vi "Autonomous Independent.vi"   [LabVIEW 2017] (continued)
                          n864 = call "PID Distance.vi"("Distance"=26.0, "Angle"=w3022, "RightEncoder"=w3027, "LeftEncoder"=w3028, "GyroDevRef"=w3029, "RobotDriveDevRef"=w3030) -> ("RightEncoder 2"=w3023:T11, "LeftEncoder 2"=w3024:T11, "GyroDevRef 2"=w3025:T8, "RobotDriveDevRef 2"=w3026:T1)  [unwired: 2 in]
                        }
                        frame #4 {
                          n865 = global write "Robot Global Data.vi" "Current State"(TRUE ("Current State")) -> ()
                          n866 = Wait (ms)(milliseconds to wait=u32 500) -> ()  [unwired: 1 out]
                        }
                        frame #5 {
                          n867 = global read "Robot Global Data.vi" "Axes"() -> (w3043:dbl[])
                          n868 = global write "Robot Global Data.vi" "Lift_Position"(2.0) -> ()
                          n869 = Wait (ms)(milliseconds to wait=u32 250) -> ()  [unwired: 1 out]
                          n870 = Array To Cluster(array=w3043) -> (cluster=w3042:T15)
                          n871 = Bundle By Name(cluster=w3042, "Axes[1]"=-1.0) -> (w3040:T15)
                          n872 = Cluster To Array(cluster=w3040) -> (array=w3039:dbl[])
                          n873 = global write "Robot Global Data.vi" "Axes"(w3039) -> ()
                        }
                        frame #6 {
                          n874 = global read "Robot Global Data.vi" "Tracked Angle"() -> (w3049:dbl)
                          n875 = call "PID Distance.vi"("Distance"=40.0, "Angle"=w3049, "RightEncoder"=w3050, "LeftEncoder"=w3053, "GyroDevRef"=w3052, "RobotDriveDevRef"=w3051) -> ()  [unwired: 2 in, 4 out]
                        }
                        frame #7 {
                          n876 = global read "Robot Global Data.vi" "Axes"() -> (w3060:dbl[])
                          n877 = Wait (ms)(milliseconds to wait=u32 250) -> ()  [unwired: 1 out]
                          n878 = Array To Cluster(array=w3060) -> (cluster=w3059:T15)
                          n879 = Bundle By Name(cluster=w3059, "Axes[1]"=1.0) -> (w3057:T15)
                          n880 = Cluster To Array(cluster=w3057) -> (array=w3056:dbl[])
                          n881 = global write "Robot Global Data.vi" "Axes"(w3056) -> ()
                        }
                        frame #8 {
                          n882 = global write "Robot Global Data.vi" "Current State"(FALSE ("Current State")) -> ()
                        }
                      }
                    }
                    frame Default {
                    }
                  }
                }
              }
            }
            frame "L" {
              n883 = flat-sequence {
                tunnel: [w3127] -> w3115
                tunnel: [w3126] -> w3116
                tunnel: [w3124] -> w3117
                tunnel: [w3125] -> w3118
                tunnel: w3074 -> [w3123]
                tunnel: w3073 -> [w3122]
                tunnel: w3072 -> [w3121]
                tunnel: w3071 -> [w3120]
                tunnel: [w3148] -> w3114
                tunnel: w3118 -> [w3144]
                tunnel: w3117 -> [w3145]
                tunnel: w3116 -> [w3147]
                tunnel: w3115 -> [w3149]
                tunnel: [w3146] -> w3113
                tunnel: [w3145] -> w3112
                tunnel: [w3144] -> w3111
                tunnel: w3114 -> [w3159]
                tunnel: [w3159] -> w3110
                tunnel: w3113 -> [w3158]
                tunnel: [w3158] -> w3109
                tunnel: [w3157] -> w3108
                tunnel: [w3156] -> w3107
                tunnel: w3112 -> [w3154]
                tunnel: w3111 -> [w3153]
                tunnel: w3110 -> [w3165]
                tunnel: [w3163] -> w3106
                tunnel: w3109 -> [w3164]
                tunnel: [w3162] -> w3105
                tunnel: w3108 -> [w3167]
                tunnel: w3107 -> [w3166]
                tunnel: [w3161] -> w3104
                tunnel: [w3160] -> w3103
                tunnel: w3106 -> [w3174]
                tunnel: [w3173] -> w3102
                tunnel: [w3172] -> w3101
                tunnel: w3105 -> [w3172]
                tunnel: [w3171] -> w3100
                tunnel: w3104 -> [w3171]
                tunnel: [w3170] -> w3099
                tunnel: w3103 -> [w3170]
                tunnel: [w3185] -> w3098
                tunnel: w3102 -> [w3185]
                tunnel: [w3184] -> w3097
                tunnel: w3101 -> [w3184]
                tunnel: [w3183] -> w3096
                tunnel: w3100 -> [w3183]
                tunnel: [w3182] -> w3095
                tunnel: w3099 -> [w3182]
                tunnel: w3098 -> [w3190]
                tunnel: w3097 -> [w3191]
                tunnel: [w3191] -> w3094
                tunnel: [w3190] -> w3093
                tunnel: [w3189] -> w3092
                tunnel: w3096 -> [w3189]
                tunnel: [w3188] -> w3091
                tunnel: w3095 -> [w3188]
                tunnel: [w3204] -> w3090
                tunnel: w3094 -> [w3206]
                tunnel: w3093 -> [w3205]
                tunnel: w3092 -> [w3201]
                tunnel: w3091 -> [w3200]
                tunnel: [w3199] -> w3089
                tunnel: [w3198] -> w3088
                tunnel: [w3197] -> w3087
                tunnel: w3090 -> [w3213]
                tunnel: w3089 -> [w3212]
                tunnel: [w3211] -> w3069
                tunnel: w3088 -> [w3211]
                tunnel: [w3210] -> w3067
                tunnel: w3087 -> [w3210]
                tunnel: [w3209] -> w3065
                tunnel: [w3208] -> w3063
                tunnel: w3069 -> [w3220]
                tunnel: [w3216] -> w3068
                tunnel: w3067 -> [w3219]
                tunnel: [w3215] -> w3066
                tunnel: w3065 -> [w3222]
                tunnel: [w3218] -> w3064
                tunnel: w3063 -> [w3221]
                tunnel: [w3217] -> w3062
                tunnel: w3068 -> [w3248]
                tunnel: w3066 -> [w3247]
                tunnel: [w3245] -> w3086
                tunnel: w3064 -> [w3245]
                tunnel: [w3244] -> w3085
                tunnel: w3062 -> [w3244]
                tunnel: [w3243] -> w3084
                tunnel: [w3242] -> w3083
                tunnel: w3086 -> [w3263]
                tunnel: w3085 -> [w3262]
                tunnel: w3084 -> [w3261]
                tunnel: w3083 -> [w3260]
                tunnel: [w3259] -> w3082
                tunnel: [w3258] -> w3081
                tunnel: [w3257] -> w3080
                tunnel: [w3256] -> w3079
                tunnel: [w3268] -> w3078
                tunnel: [w3265] -> w3077
                tunnel: [w3267] -> w3076
                tunnel: [w3266] -> w3075
                tunnel: w3079 -> [w3265]
                tunnel: w3080 -> [w3266]
                tunnel: w3081 -> [w3267]
                tunnel: w3082 -> [w3268]
                tunnel: w3078 -> [w3275]
                tunnel: w3077 -> [w3274]
                tunnel: w3076 -> [w3273]
                tunnel: w3075 -> [w3272]
                tunnel: w3070 -> [w3271]
                frame #0 {
                  n884 = while {
                    tunnel: [w3133] -> w3119
                    stop <- w3132 stop-if-true
                    w3136 = 100.0 ("y")
                    w3139 = 20.0 ("y")
                    n885 = Wait (ms)(milliseconds to wait=u32 10) -> ()  [unwired: 1 out]
                    n886 = global read "Robot Global Data.vi" "Distance 2"() -> (w3134:dbl)
                    n887 = global read "Robot Global Data.vi" "Distance"() -> (w3135:dbl)
                    n888 = Greater?(x=w3135, y=w3139) -> (0:w3141:bool)
                    n889 = Greater?(x=w3134, y=w3139) -> (0:w3140:bool)
                    n890 = Greater?(x=w3135, y=w3136) -> (0:w3138:bool)
                    n891 = Greater?(x=w3134, y=w3136) -> (0:w3137:bool)
                    n892 = Or(x=w3141, y=w3140) -> (x .or. y?=w3130:bool)
                    n893 = Or(x=w3138, y=w3137) -> (x .or. y?=w3132:bool)
                    n894 = global write "Robot Global Data.vi" "Raise_Mast"(w3130) -> ()
                    n895 = case shown="True" w3132 {
                      tunnel: [0.0 2.0] -> w3133
                      frame False {
                      }
                      frame True {
                      }
                    }
                  }
                  n896 = call "PID Distance.vi"("Distance"=295.0, "Angle"=-2.0, "RightEncoder"=w3120, "LeftEncoder"=w3121, "GyroDevRef"=w3122, "RobotDriveDevRef"=w3123) -> ("RightEncoder 2"=w3124:T11, "LeftEncoder 2"=w3125:T11, "GyroDevRef 2"=w3126:T8, "RobotDriveDevRef 2"=w3127:T1)  [unwired: 2 in]
                  n897 = global write "Robot Global Data.vi" "Lift_Position"(w3119) -> ()
                }
                frame #1 {
                  n898 = call "PID turning.vi"("Angle"=90.0, "GyroDevRef"=w3147, "RobotDriveDevRef"=w3149) -> ("GyroDevRef 2"=w3146:T8, "RobotDriveDevRef 2"=w3148:T1)  [unwired: 7 in]
                  n899 = global write "Robot Global Data.vi" "Lift_Position"(3.0) -> ()
                  n900 = global write "Robot Global Data.vi" "Raise_Mast"(TRUE ("Current State")) -> ()
                }
                frame #2 {
                  n901 = call <vilib>:"WPI_EncoderReset.vi"("EncoderDevRef"=w3153) -> ("EncoderDevRef"=w3156:T11)  [unwired: 9 in, 1 out]
                  n902 = Wait (ms)(milliseconds to wait=u32 100) -> ()  [unwired: 1 out]
                  n903 = call <vilib>:"WPI_EncoderReset.vi"("EncoderDevRef"=w3154) -> ("EncoderDevRef"=w3157:T11)  [unwired: 9 in, 1 out]
                }
                frame #3 {
                  n904 = call "PID Distance.vi"("Distance"=25.0, "Angle"=90.0, "RightEncoder"=w3167, "LeftEncoder"=w3166, "GyroDevRef"=w3164, "RobotDriveDevRef"=w3165) -> ("RightEncoder 2"=w3160:T11, "LeftEncoder 2"=w3161:T11, "GyroDevRef 2"=w3162:T8, "RobotDriveDevRef 2"=w3163:T1)  [unwired: 2 in]
                }
                frame #4 {
                  w3175 = 0.0 ("Left axis value")
                  n905 = global read "Robot Global Data.vi" "Axes"() -> (w3178:dbl[])
                  n906 = Wait (ms)(milliseconds to wait=u32 500) -> ()  [unwired: 1 out]
                  n907 = Array To Cluster(array=w3178) -> (cluster=w3177:T15)
                  n908 = Bundle By Name(cluster=w3177, "Axes[1]"=0.25) -> (w3180:T15)
                  n909 = Cluster To Array(cluster=w3180) -> (array=w3179:dbl[])
                  n910 = call <vilib>:"WPI_RobotDriveTankDrive.vi"("Right axis value"=w3175, "Left axis value"=w3175, "RobotDriveDevRef"=w3174) -> ("RobotDriveDevRef"=w3173:T1)  [unwired: 6 in, 2 out]
                  n911 = global write "Robot Global Data.vi" "Axes"(w3179) -> ()
                }
                frame #5 {
                  n912 = global write "Robot Global Data.vi" "Current State"(FALSE ("Current State")) -> ()
                  n913 = Wait (ms)(milliseconds to wait=u32 400) -> ()  [unwired: 1 out]
                }
                frame #6 {
                  n914 = global read "Robot Global Data.vi" "Axes"() -> (w3193:dbl[])
                  n915 = Array To Cluster(array=w3193) -> (cluster=w3192:T15)
                  n916 = Bundle By Name(cluster=w3192, "Axes[1]"=-1.0) -> (w3195:T15)
                  n917 = Cluster To Array(cluster=w3195) -> (array=w3194:dbl[])
                  n918 = global write "Robot Global Data.vi" "Axes"(w3194) -> ()
                }
                frame #7 {
                  n919 = call "PID Distance.vi"("Distance"=7.0, "Angle"=90.0, "RightEncoder"=w3200, "LeftEncoder"=w3201, "GyroDevRef"=w3206, "RobotDriveDevRef"=w3205) -> ("RightEncoder 2"=w3197:T11, "LeftEncoder 2"=w3198:T11, "GyroDevRef 2"=w3199:T8, "RobotDriveDevRef 2"=w3204:T1)  [unwired: 2 in]
                }
                frame #8 {
                  n920 = global write "Robot Global Data.vi" "Lift_Position"(1.0) -> ()
                  n921 = call "PID turning.vi"("Angle"=155.0, "GyroDevRef"=w3212, "RobotDriveDevRef"=w3213) -> ("GyroDevRef 2"=w3208:T8, "RobotDriveDevRef 2"=w3209:T1)  [unwired: 7 in]
                }
                frame #9 {
                  n922 = global read "Robot Global Data.vi" "PIXY Output"() -> (w3226:T16)
                  n923 = Unbundle By Name(w3226) -> ("SIGNATURE NUMBER"=w3225:u16)
                  n924 = global read "Robot Global Data.vi" "Cube Signature"() -> (w3224:dbl)
                  n925 = Equal?(x=w3225, y=w3224) -> (x = y?=w3223:bool)
                  n926 = case shown="False" w3223 {
                    tunnel: [w3233 w3237] -> w3215
                    tunnel: [w3232 w3238] -> w3216
                    tunnel: [w3231 w3239] -> w3217
                    tunnel: [w3235 w3240] -> w3218
                    tunnel: w3220 -> [w3232 w3238]
                    tunnel: w3219 -> [w3233 w3237]
                    tunnel: w3221 -> [w3234 w3239]
                    tunnel: w3222 -> [w3236 w3240]
                    frame True {
                      n927 = call <vilib>:"WPI_GyroGetAngle.vi"("GyroDevRef"=w3234) -> ("Angle"=w3230:dbl, "GyroDevRef"=w3231:T8)  [unwired: 6 in, 3 out]
                      n928 = In Range and Coerce(upper limit=170.0, x=w3230, lower limit=155.0) -> (coerced(x)=w3229:dbl)  [unwired: 1 out]
                      n929 = global write "Robot Global Data.vi" "Tracked Angle"(w3229) -> ()
                      n930 = call "PID vision.vi"("RobotDriveDevRef in"=w3236) -> ("RobotDriveDevRef out"=w3235:T1)  [unwired: 9 in, 1 out]
                    }
                    frame False {
                      n931 = global write "Robot Global Data.vi" "Tracked Angle"(155.0) -> ()
                    }
                  }
                }
                frame #10 {
                  n932 = call <vilib>:"WPI_EncoderReset.vi"("EncoderDevRef"=w3248) -> ("EncoderDevRef"=w3243:T11)  [unwired: 9 in, 1 out]
                  n933 = Wait (ms)(milliseconds to wait=u32 10) -> ()  [unwired: 1 out]
                  n934 = call <vilib>:"WPI_EncoderReset.vi"("EncoderDevRef"=w3247) -> ("EncoderDevRef"=w3242:T11)  [unwired: 9 in, 1 out]
                }
                frame #11 {
                  n935 = global write "Robot Global Data.vi" "Lift_Position"(0.0) -> ()
                  n936 = global read "Robot Global Data.vi" "Axes"() -> (w3253:dbl[])
                  n937 = Array To Cluster(array=w3253) -> (cluster=w3252:T15)
                  n938 = global read "Robot Global Data.vi" "Tracked Angle"() -> (w3250:dbl)
                  n939 = Bundle By Name(cluster=w3252, "Axes[1]"=1.0) -> (w3255:T15)
                  n940 = call "PID Distance.vi"("Distance"=106.0, "Angle"=w3250, "RightEncoder"=w3260, "LeftEncoder"=w3261, "GyroDevRef"=w3262, "RobotDriveDevRef"=w3263) -> ("RightEncoder 2"=w3256:T11, "LeftEncoder 2"=w3257:T11, "GyroDevRef 2"=w3258:T8, "RobotDriveDevRef 2"=w3259:T1)  [unwired: 2 in]
                  n941 = Cluster To Array(cluster=w3255) -> (array=w3254:dbl[])
                  n942 = global write "Robot Global Data.vi" "Axes"(w3254) -> ()
                }
                frame #12 {
                  n943 = global write "Robot Global Data.vi" "Current State"(TRUE ("Current State")) -> ()
                  n944 = Wait (ms)(milliseconds to wait=u32 750) -> ()  [unwired: 1 out]
                }
                frame #13 {
                  n945 = case shown="\"R\"" w3271 {
                    tunnel: w3275 -> [w3279 w3332 _]
                    tunnel: w3274 -> [w3276 w3331 _]
                    tunnel: w3273 -> [w3278 w3330 _]
                    tunnel: w3272 -> [w3277 w3329 _]
                    frame "L" {
                      n946 = flat-sequence {
                        tunnel: w3279 -> [w3291]
                        tunnel: w3278 -> [w3290]
                        tunnel: w3276 -> [w3288]
                        tunnel: w3277 -> [w3289]
                        frame #0 {
                          n947 = global read "Robot Global Data.vi" "Axes"() -> (w3284:dbl[])
                          n948 = global write "Robot Global Data.vi" "Lift_Position"(2.0) -> ()
                          n949 = Wait (ms)(milliseconds to wait=u32 250) -> ()  [unwired: 1 out]
                          n950 = Array To Cluster(array=w3284) -> (cluster=w3283:T15)
                          n951 = Bundle By Name(cluster=w3283, "Axes[1]"=-1.0) -> (w3286:T15)
                          n952 = Cluster To Array(cluster=w3286) -> (array=w3285:dbl[])
                          n953 = global write "Robot Global Data.vi" "Axes"(w3285) -> ()
                        }
                        frame #1 {
                          n954 = global read "Robot Global Data.vi" "Tracked Angle"() -> (w3287:dbl)
                          n955 = call "PID Distance.vi"("Distance"=119.0, "Angle"=w3287, "RightEncoder"=w3288, "LeftEncoder"=w3289, "GyroDevRef"=w3290, "RobotDriveDevRef"=w3291) -> ()  [unwired: 2 in, 4 out]
                        }
                        frame #2 {
                          n956 = global read "Robot Global Data.vi" "Axes"() -> (w3296:dbl[])
                          n957 = Wait (ms)(milliseconds to wait=u32 200) -> ()  [unwired: 1 out]
                          n958 = Array To Cluster(array=w3296) -> (cluster=w3295:T15)
                          n959 = Bundle By Name(cluster=w3295, "Axes[1]"=0.5) -> (w3298:T15)
                          n960 = Cluster To Array(cluster=w3298) -> (array=w3297:dbl[])
                          n961 = global write "Robot Global Data.vi" "Axes"(w3297) -> ()
                        }
                        frame #3 {
                          n962 = global write "Robot Global Data.vi" "Current State"(FALSE ("Current State")) -> ()
                          n963 = Wait (ms)(milliseconds to wait=u32 500) -> ()  [unwired: 1 out]
                        }
                      }
                    }
                    frame "R" {
                      n964 = flat-sequence {
                        tunnel: w3332 -> [w3343]
                        tunnel: w3331 -> [w3348]
                        tunnel: w3330 -> [w3342]
                        tunnel: w3329 -> [w3341]
                        tunnel: [w3347] -> w3328
                        tunnel: [w3346] -> w3327
                        tunnel: [w3345] -> w3325
                        tunnel: [w3344] -> w3323
                        tunnel: w3328 -> [w3356]
                        tunnel: w3327 -> [w3355]
                        tunnel: [w3354] -> w3326
                        tunnel: w3325 -> [w3354]
                        tunnel: [w3353] -> w3324
                        tunnel: w3323 -> [w3353]
                        tunnel: [w3352] -> w3321
                        tunnel: [w3351] -> w3319
                        tunnel: w3326 -> [w3363]
                        tunnel: w3324 -> [w3362]
                        tunnel: [w3361] -> w3322
                        tunnel: w3321 -> [w3361]
                        tunnel: [w3360] -> w3320
                        tunnel: w3319 -> [w3360]
                        tunnel: [w3359] -> w3318
                        tunnel: [w3358] -> w3317
                        tunnel: w3322 -> [w3373]
                        tunnel: w3320 -> [w3372]
                        tunnel: w3318 -> [w3371]
                        tunnel: w3317 -> [w3370]
                        tunnel: [w3369] -> w3316
                        tunnel: [w3368] -> w3315
                        tunnel: [w3366] -> w3314
                        tunnel: [w3365] -> w3313
                        tunnel: [w3379] -> w3312
                        tunnel: [w3378] -> w3311
                        tunnel: [w3377] -> w3310
                        tunnel: [w3376] -> w3309
                        tunnel: w3313 -> [w3376]
                        tunnel: w3314 -> [w3377]
                        tunnel: w3315 -> [w3378]
                        tunnel: w3316 -> [w3379]
                        tunnel: [w3389] -> w3302
                        tunnel: w3312 -> [w3389]
                        tunnel: [w3388] -> w3304
                        tunnel: w3311 -> [w3388]
                        tunnel: [w3387] -> w3306
                        tunnel: w3310 -> [w3387]
                        tunnel: [w3386] -> w3308
                        tunnel: w3309 -> [w3386]
                        tunnel: w3308 -> [w3401]
                        tunnel: [w3401] -> w3307
                        tunnel: w3306 -> [w3400]
                        tunnel: [w3400] -> w3305
                        tunnel: w3304 -> [w3399]
                        tunnel: [w3399] -> w3303
                        tunnel: w3302 -> [w3398]
                        tunnel: [w3398] -> w3301
                        tunnel: w3307 -> [w3402]
                        tunnel: w3305 -> [w3403]
                        tunnel: w3303 -> [w3404]
                        tunnel: w3301 -> [w3405]
                        frame #0 {
                          n965 = global read "Robot Global Data.vi" "Axes"() -> (w3337:dbl[])
                          n966 = global write "Robot Global Data.vi" "Lift_Position"(2.0) -> ()
                          n967 = Wait (ms)(milliseconds to wait=u32 250) -> ()  [unwired: 1 out]
                          n968 = Array To Cluster(array=w3337) -> (cluster=w3336:T15)
                          n969 = Bundle By Name(cluster=w3336, "Axes[1]"=-1.0) -> (w3339:T15)
                          n970 = Cluster To Array(cluster=w3339) -> (array=w3338:dbl[])
                          n971 = global write "Robot Global Data.vi" "Axes"(w3338) -> ()
                        }
                        frame #1 {
                          n972 = global read "Robot Global Data.vi" "Tracked Angle"() -> (w3340:dbl)
                          n973 = call "PID Distance.vi"("Distance"=-20.0, "Angle"=w3340, "RightEncoder"=w3348, "LeftEncoder"=w3341, "GyroDevRef"=w3342, "RobotDriveDevRef"=w3343) -> ("RightEncoder 2"=w3344:T11, "LeftEncoder 2"=w3345:T11, "GyroDevRef 2"=w3346:T8, "RobotDriveDevRef 2"=w3347:T1)  [unwired: 2 in]
                        }
                        frame #2 {
                          n974 = call "PID turning.vi"("Angle"=90.0, "GyroDevRef"=w3355, "RobotDriveDevRef"=w3356) -> ("GyroDevRef 2"=w3351:T8, "RobotDriveDevRef 2"=w3352:T1)  [unwired: 7 in]
                          n975 = global write "Robot Global Data.vi" "Lift_Position"(3.0) -> ()
                        }
                        frame #3 {
                          n976 = call <vilib>:"WPI_EncoderReset.vi"("EncoderDevRef"=w3363) -> ("EncoderDevRef"=w3359:T11)  [unwired: 9 in, 1 out]
                          n977 = Wait (ms)(milliseconds to wait=u32 10) -> ()  [unwired: 1 out]
                          n978 = call <vilib>:"WPI_EncoderReset.vi"("EncoderDevRef"=w3362) -> ("EncoderDevRef"=w3358:T11)  [unwired: 9 in, 1 out]
                        }
                        frame #4 {
                          n979 = call "PID Distance.vi"("Distance"=30.0, "Angle"=90.0, "RightEncoder"=w3370, "LeftEncoder"=w3371, "GyroDevRef"=w3372, "RobotDriveDevRef"=w3373) -> ("RightEncoder 2"=w3365:T11, "LeftEncoder 2"=w3366:T11, "GyroDevRef 2"=w3368:T8, "RobotDriveDevRef 2"=w3369:T1)  [unwired: 2 in]
                          n980 = global write "Robot Global Data.vi" "Lift_Position"(3.0) -> ()
                        }
                        frame #5 {
                          n981 = global read "Robot Global Data.vi" "Axes"() -> (w3383:dbl[])
                          n982 = Wait (ms)(milliseconds to wait=u32 500) -> ()  [unwired: 1 out]
                          n983 = Array To Cluster(array=w3383) -> (cluster=w3382:T15)
                          n984 = Bundle By Name(cluster=w3382, "Axes[1]"=0.3) -> (w3385:T15)
                          n985 = Cluster To Array(cluster=w3385) -> (array=w3384:dbl[])
                          n986 = global write "Robot Global Data.vi" "Axes"(w3384) -> ()
                        }
                        frame #6 {
                          n987 = global write "Robot Global Data.vi" "Current State"(FALSE ("Current State")) -> ()
                          n988 = Wait (ms)(milliseconds to wait=u32 400) -> ()  [unwired: 1 out]
                        }
                        frame #7 {
                          n989 = global read "Robot Global Data.vi" "Axes"() -> (w3395:dbl[])
                          n990 = Wait (ms)(milliseconds to wait=u32 250) -> ()  [unwired: 1 out]
                          n991 = Array To Cluster(array=w3395) -> (cluster=w3394:T15)
                          n992 = Bundle By Name(cluster=w3394, "Axes[1]"=-1.0) -> (w3397:T15)
                          n993 = Cluster To Array(cluster=w3397) -> (array=w3396:dbl[])
                          n994 = global write "Robot Global Data.vi" "Axes"(w3396) -> ()
                        }
                        frame #8 {
                          n995 = call "PID Distance.vi"("Distance"=0.0, "Angle"=-90.0, "RightEncoder"=w3402, "LeftEncoder"=w3403, "GyroDevRef"=w3404, "RobotDriveDevRef"=w3405) -> ()  [unwired: 2 in, 4 out]
                        }
                        frame #9 {
                          n996 = global write "Robot Global Data.vi" "Lift_Position"(1.0) -> ()
                        }
                      }
                    }
                    frame Default {
                    }
                  }
                }
              }
            }
            frame Default {
              n997 = flat-sequence {
                tunnel: w3410 -> [w3418]
                tunnel: w3409 -> [w3417]
                tunnel: w3411 -> [w3415]
                tunnel: [w3416] -> w3413
                tunnel: w3412 -> [w3414]
                tunnel: w3413 -> [w3421]
                frame #0 {
                  n998 = call "PID Distance.vi"("Distance"=90.0, "Angle"=0.0, "RightEncoder"=w3414, "LeftEncoder"=w3415, "GyroDevRef"=w3417, "RobotDriveDevRef"=w3418) -> ("RobotDriveDevRef 2"=w3416:T1)  [unwired: 2 in, 3 out]
                }
                frame #1 {
                  w3422 = 0.0
                  n999 = call <vilib>:"WPI_RobotDriveTankDrive.vi"("Right axis value"=w3422, "Left axis value"=w3422, "RobotDriveDevRef"=w3421) -> ()  [unwired: 6 in, 3 out]
                }
              }
            }
          }
        }
      }
    }
    frame "Left Scale V2" {
      n1000 = flat-sequence {
        tunnel: w3430 -> [w3459]
        tunnel: w3428 -> [w3457]
        tunnel: w3429 -> [w3456]
        tunnel: [w3455] -> w3434
        tunnel: [w3454] -> w3433
        tunnel: [w3453] -> w3432
        tunnel: [w3452] -> w3431
        tunnel: w3426 -> [w3445]
        tunnel: w3427 -> [w3435]
        tunnel: w3425 -> [w3462]
        tunnel: w3434 -> [w3466]
        tunnel: w3433 -> [w3465]
        tunnel: w3432 -> [w3464]
        tunnel: w3431 -> [w3463]
        tunnel: w3424 -> [w3461]
        tunnel: w3423 -> [w3460]
        frame #0 {
          w3458 = 0.0 ("Left axis value")
          n1001 = global read "Robot Global Data.vi" "Axes"() -> (w3438:dbl[])
          n1002 = Multiply(x=w3445, y=1000.0) -> (x*y=w3446:dbl)
          n1003 = global write "Robot Global Data.vi" "Lift_Position"(0.0) -> ()
          n1004 = global write "Robot Global Data.vi" "Raise_Mast"(FALSE ("Current State")) -> ()
          n1005 = global write "Robot Global Data.vi" "Current State"(TRUE ("Current State")) -> ()
          n1006 = Wait (ms)(milliseconds to wait=u32 100) -> ()  [unwired: 1 out]
          n1007 = Array To Cluster(array=w3438) -> (cluster=w3437:T15)
          n1008 = Bundle By Name(cluster=w3437, "Axes[1]"=-1.0) -> (w3440:T15)
          n1009 = Greater?(x=w3446, y=11000.0) -> (0:w3448:bool)
          n1010 = Equal?(x=w3446, y=0.0) -> (x = y?=w3449:bool)
          n1011 = Or(x=w3448, y=w3449) -> ()  [unwired: 1 out]
          n1012 = Cluster To Array(cluster=w3440) -> (array=w3439:dbl[])
          n1013 = call <vilib>:"WPI_GyroReset.vi"("GyroDevRef"=w3456) -> ("GyroDevRef"=w3452:T8)  [unwired: 9 in, 1 out]
          n1014 = call <vilib>:"WPI_EncoderReset.vi"("EncoderDevRef"=w3435) -> ("EncoderDevRef"=w3454:T11)  [unwired: 9 in, 1 out]
          n1015 = global write "Robot Global Data.vi" "Axes"(w3439) -> ()
          n1016 = call <vilib>:"WPI_EncoderReset.vi"("EncoderDevRef"=w3457) -> ("EncoderDevRef"=w3453:T11)  [unwired: 9 in, 1 out]
          n1017 = call <vilib>:"WPI_RobotDriveTankDrive.vi"("Right axis value"=w3458, "Left axis value"=w3458, "RobotDriveDevRef"=w3459) -> ("RobotDriveDevRef"=w3455:T1)  [unwired: 6 in, 2 out]
        }
        frame #1 {
          n1018 = case shown="\"L\"" w3462 {
            tunnel: w3466 -> [w3469 w3870 w4221]
            tunnel: w3465 -> [w3472 w3867 w4223]
            tunnel: w3464 -> [w3471 w3868 w4222]
            tunnel: w3463 -> [w3470 w3869 w4220]
            tunnel: w3461 -> [w3468 w3866 _]
            tunnel: w3460 -> [w3467 w3857 _]
            frame "R" {
              n1019 = flat-sequence {
                tunnel: [w3532] -> w3524
                tunnel: [w3531] -> w3523
                tunnel: [w3529] -> w3522
                tunnel: [w3530] -> w3521
                tunnel: w3472 -> [w3525]
                tunnel: w3471 -> [w3526]
                tunnel: w3470 -> [w3527]
                tunnel: w3469 -> [w3528]
                tunnel: w3524 -> [w3543]
                tunnel: w3523 -> [w3544]
                tunnel: [w3547] -> w3520
                tunnel: w3522 -> [w3547]
                tunnel: [w3546] -> w3519
                tunnel: w3521 -> [w3546]
                tunnel: [w3541] -> w3518
                tunnel: [w3542] -> w3517
                tunnel: w3520 -> [w3554]
                tunnel: w3519 -> [w3553]
                tunnel: [w3552] -> w3516
                tunnel: [w3551] -> w3515
                tunnel: [w3550] -> w3514
                tunnel: w3518 -> [w3550]
                tunnel: [w3548] -> w3513
                tunnel: w3517 -> [w3548]
                tunnel: w3516 -> [w3559]
                tunnel: w3515 -> [w3560]
                tunnel: w3514 -> [w3561]
                tunnel: [w3557] -> w3512
                tunnel: [w3558] -> w3511
                tunnel: w3513 -> [w3562]
                tunnel: [w3555] -> w3510
                tunnel: [w3556] -> w3509
                tunnel: w3512 -> [w3574]
                tunnel: w3511 -> [w3573]
                tunnel: [w3572] -> w3508
                tunnel: [w3571] -> w3507
                tunnel: [w3577] -> w3506
                tunnel: w3510 -> [w3577]
                tunnel: [w3576] -> w3505
                tunnel: w3509 -> [w3576]
                tunnel: w3508 -> [w3583]
                tunnel: [w3583] -> w3504
                tunnel: [w3582] -> w3503
                tunnel: [w3581] -> w3502
                tunnel: [w3580] -> w3501
                tunnel: w3507 -> [w3580]
                tunnel: w3506 -> [w3579]
                tunnel: w3505 -> [w3578]
                tunnel: w3504 -> [w3591]
                tunnel: [w3588] -> w3500
                tunnel: w3503 -> [w3590]
                tunnel: w3502 -> [w3589]
                tunnel: w3501 -> [w3592]
                tunnel: [w3587] -> w3499
                tunnel: [w3586] -> w3498
                tunnel: [w3585] -> w3497
                tunnel: w3500 -> [w3599]
                tunnel: [w3598] -> w3496
                tunnel: w3499 -> [w3596]
                tunnel: [w3595] -> w3495
                tunnel: w3498 -> [w3601]
                tunnel: [w3601] -> w3494
                tunnel: w3497 -> [w3600]
                tunnel: [w3600] -> w3493
                tunnel: w3496 -> [w3612]
                tunnel: [w3606] -> w3492
                tunnel: [w3605] -> w3491
                tunnel: w3495 -> [w3605]
                tunnel: [w3604] -> w3490
                tunnel: w3494 -> [w3604]
                tunnel: [w3603] -> w3489
                tunnel: w3493 -> [w3603]
                tunnel: w3492 -> [w3619]
                tunnel: [w3619] -> w3488
                tunnel: w3491 -> [w3618]
                tunnel: [w3618] -> w3487
                tunnel: w3490 -> [w3617]
                tunnel: [w3617] -> w3486
                tunnel: w3489 -> [w3616]
                tunnel: [w3616] -> w3485
                tunnel: w3488 -> [w3623]
                tunnel: [w3621] -> w3484
                tunnel: w3487 -> [w3622]
                tunnel: [w3620] -> w3483
                tunnel: w3486 -> [w3626]
                tunnel: [w3626] -> w3482
                tunnel: w3485 -> [w3625]
                tunnel: [w3625] -> w3481
                tunnel: w3484 -> [w3639]
                tunnel: w3483 -> [w3638]
                tunnel: w3482 -> [w3637]
                tunnel: w3481 -> [w3636]
                tunnel: [w3630] -> w3480
                tunnel: [w3629] -> w3479
                tunnel: [w3628] -> w3478
                tunnel: [w3627] -> w3477
                tunnel: w3480 -> [w3646]
                tunnel: [w3646] -> w3476
                tunnel: w3479 -> [w3645]
                tunnel: [w3645] -> w3475
                tunnel: w3478 -> [w3644]
                tunnel: [w3644] -> w3474
                tunnel: w3477 -> [w3643]
                tunnel: [w3643] -> w3473
                tunnel: w3476 -> [w3652]
                tunnel: w3475 -> [w3651]
                tunnel: w3474 -> [w3649]
                tunnel: w3473 -> [w3650]
                tunnel: w3468 -> [w3648]
                tunnel: w3467 -> [w3647]
                frame #0 {
                  n1020 = while {
                    stop <- w3535 stop-if-true
                    w3536 = 20.0 ("y")
                    n1021 = global read "Robot Global Data.vi" "Distance 2"() -> (w3537:dbl)
                    n1022 = global read "Robot Global Data.vi" "Distance"() -> (w3538:dbl)
                    n1023 = Greater?(x=w3538, y=w3536) -> (0:w3540:bool)
                    n1024 = Greater?(x=w3537, y=w3536) -> (0:w3539:bool)
                    n1025 = And(x=w3540, y=w3539) -> (x .and. y?=w3535:bool)
                    n1026 = global write "Robot Global Data.vi" "Raise_Mast"(w3535) -> ()
                  }
                  n1027 = call "PID Distance.vi"("Distance"=225.0, "Angle"=0.0, "RightEncoder"=w3525, "LeftEncoder"=w3526, "GyroDevRef"=w3527, "RobotDriveDevRef"=w3528) -> ("RightEncoder 2"=w3529:T11, "LeftEncoder 2"=w3530:T11, "GyroDevRef 2"=w3531:T8, "RobotDriveDevRef 2"=w3532:T1)  [unwired: 2 in]
                }
                frame #1 {
                  n1028 = call "PID turning.vi"("Angle"=90.0, "GyroDevRef"=w3544, "RobotDriveDevRef"=w3543) -> ("GyroDevRef 2"=w3541:T8, "RobotDriveDevRef 2"=w3542:T1)  [unwired: 7 in]
                }
                frame #2 {
                  n1029 = call <vilib>:"WPI_EncoderReset.vi"("EncoderDevRef"=w3553) -> ("EncoderDevRef"=w3551:T11)  [unwired: 9 in, 1 out]
                  n1030 = Wait (ms)(milliseconds to wait=u32 10) -> ()  [unwired: 1 out]
                  n1031 = call <vilib>:"WPI_EncoderReset.vi"("EncoderDevRef"=w3554) -> ("EncoderDevRef"=w3552:T11)  [unwired: 9 in, 1 out]
                }
                frame #3 {
                  n1032 = global read "Robot Global Data.vi" "Axes"() -> (w3566:dbl[])
                  n1033 = call "PID Distance.vi"("Distance"=199.0, "Angle"=90.0, "RightEncoder"=w3559, "LeftEncoder"=w3560, "GyroDevRef"=w3561, "RobotDriveDevRef"=w3562) -> ("RightEncoder 2"=w3556:T11, "LeftEncoder 2"=w3555:T11, "GyroDevRef 2"=w3558:T8, "RobotDriveDevRef 2"=w3557:T1)  [unwired: 2 in]
                  n1034 = global write "Robot Global Data.vi" "Lift_Position"(2.0) -> ()
                  n1035 = Array To Cluster(array=w3566) -> (cluster=w3565:T15)
                  n1036 = Bundle By Name(cluster=w3565, "Axes[1]"=-1.0) -> (w3564:T15)
                  n1037 = Cluster To Array(cluster=w3564) -> (array=w3563:dbl[])
                  n1038 = global write "Robot Global Data.vi" "Axes"(w3563) -> ()
                }
                frame #4 {
                  n1039 = call "PID turning.vi"("Angle"=0.0, "GyroDevRef"=w3573, "RobotDriveDevRef"=w3574) -> ("GyroDevRef 2"=w3571:T8, "RobotDriveDevRef 2"=w3572:T1)  [unwired: 7 in]
                }
                frame #5 {
                  n1040 = call <vilib>:"WPI_EncoderReset.vi"("EncoderDevRef"=w3579) -> ("EncoderDevRef"=w3582:T11)  [unwired: 9 in, 1 out]
                  n1041 = call <vilib>:"WPI_EncoderReset.vi"("EncoderDevRef"=w3578) -> ("EncoderDevRef"=w3581:T11)  [unwired: 9 in, 1 out]
                }
                frame #6 {
                  n1042 = call "PID Distance.vi"("Distance"=38.0, "Angle"=0.0, "RightEncoder"=w3589, "LeftEncoder"=w3590, "GyroDevRef"=w3592, "RobotDriveDevRef"=w3591) -> ("RightEncoder 2"=w3585:T11, "LeftEncoder 2"=w3586:T11, "GyroDevRef 2"=w3587:T8, "RobotDriveDevRef 2"=w3588:T1)  [unwired: 2 in]
                  n1043 = global write "Robot Global Data.vi" "Lift_Position"(3.0) -> ()
                }
                frame #7 {
                  n1044 = call "PID turning.vi"("Angle"=-20.0, "GyroDevRef"=w3596, "RobotDriveDevRef"=w3599) -> ("GyroDevRef 2"=w3595:T8, "RobotDriveDevRef 2"=w3598:T1)  [unwired: 7 in]
                }
                frame #8 {
                  w3613 = 0.0 ("Left axis value")
                  n1045 = global read "Robot Global Data.vi" "Axes"() -> (w3608:dbl[])
                  n1046 = Wait (ms)(milliseconds to wait=u32 300) -> ()  [unwired: 1 out]
                  n1047 = Array To Cluster(array=w3608) -> (cluster=w3607:T15)
                  n1048 = Bundle By Name(cluster=w3607, "Axes[1]"=0.25) -> (w3610:T15)
                  n1049 = Cluster To Array(cluster=w3610) -> (array=w3609:dbl[])
                  n1050 = call <vilib>:"WPI_RobotDriveTankDrive.vi"("Right axis value"=w3613, "Left axis value"=w3613, "RobotDriveDevRef"=w3612) -> ("RobotDriveDevRef"=w3606:T1)  [unwired: 6 in, 2 out]
                  n1051 = global write "Robot Global Data.vi" "Axes"(w3609) -> ()
                }
                frame #9 {
                  n1052 = global write "Robot Global Data.vi" "Current State"(FALSE ("Current State")) -> ()
                  n1053 = Wait (ms)(milliseconds to wait=u32 400) -> ()  [unwired: 1 out]
                }
                frame #10 {
                  n1054 = call "PID turning.vi"("Angle"=0.0, "GyroDevRef"=w3622, "RobotDriveDevRef"=w3623) -> ("GyroDevRef 2"=w3620:T8, "RobotDriveDevRef 2"=w3621:T1)  [unwired: 7 in]
                }
                frame #11 {
                  n1055 = global read "Robot Global Data.vi" "Axes"() -> (w3635:dbl[])
                  n1056 = Array To Cluster(array=w3635) -> (cluster=w3634:T15)
                  n1057 = call "PID Distance.vi"("Distance"=0.0, "Angle"=0.0, "RightEncoder"=w3636, "LeftEncoder"=w3637, "GyroDevRef"=w3638, "RobotDriveDevRef"=w3639) -> ("RightEncoder 2"=w3627:T11, "LeftEncoder 2"=w3628:T11, "GyroDevRef 2"=w3629:T8, "RobotDriveDevRef 2"=w3630:T1)  [unwired: 2 in]
                  n1058 = Bundle By Name(cluster=w3634, "Axes[1]"=-1.0) -> (w3633:T15)
                  n1059 = Cluster To Array(cluster=w3633) -> (array=w3632:dbl[])
                  n1060 = global write "Robot Global Data.vi" "Axes"(w3632) -> ()
                }
                frame #12 {
                  n1061 = global write "Robot Global Data.vi" "Lift_Position"(1.0) -> ()
                }
                frame #13 {
                  n1062 = case shown="\"R\"" w3648 {
                    tunnel: w3652 -> [w3666 w3763 _]
                    tunnel: w3651 -> [w3665 w3762 _]
                    tunnel: w3650 -> [w3664 w3759 _]
                    tunnel: w3649 -> [w3663 w3758 _]
                    tunnel: w3647 -> [w3653 w3737 _]
                    frame "L" {
                      n1063 = flat-sequence {
                        tunnel: w3666 -> [w3675]
                        tunnel: w3665 -> [w3674]
                        tunnel: [w3677] -> w3672
                        tunnel: [w3676] -> w3671
                        tunnel: w3672 -> [w3684]
                        tunnel: w3671 -> [w3683]
                        tunnel: [w3684] -> w3667
                        tunnel: [w3683] -> w3668
                        tunnel: [w3681] -> w3669
                        tunnel: [w3680] -> w3670
                        tunnel: w3664 -> [w3679]
                        tunnel: w3663 -> [w3678]
                        tunnel: w3670 -> [w3690]
                        tunnel: w3669 -> [w3691]
                        tunnel: w3668 -> [w3692]
                        tunnel: w3667 -> [w3693]
                        tunnel: [w3688] -> w3662
                        tunnel: [w3687] -> w3660
                        tunnel: [w3686] -> w3659
                        tunnel: [w3685] -> w3657
                        tunnel: w3662 -> [w3725]
                        tunnel: [w3724] -> w3661
                        tunnel: w3660 -> [w3723]
                        tunnel: w3659 -> [w3722]
                        tunnel: [w3721] -> w3658
                        tunnel: w3657 -> [w3721]
                        tunnel: [w3720] -> w3656
                        tunnel: [w3719] -> w3655
                        tunnel: [w3718] -> w3654
                        tunnel: w3661 -> [w3733]
                        tunnel: w3658 -> [w3731]
                        tunnel: w3656 -> [w3730]
                        tunnel: w3655 -> [w3729]
                        tunnel: w3654 -> [w3728]
                        tunnel: w3653 -> [w3727]
                        frame #0 {
                          n1064 = call "PID turning.vi"("Angle"=170.0, "GyroDevRef"=w3674, "RobotDriveDevRef"=w3675) -> ("GyroDevRef 2"=w3676:T8, "RobotDriveDevRef 2"=w3677:T1)  [unwired: 7 in]
                        }
                        frame #1 {
                          n1065 = call <vilib>:"WPI_EncoderReset.vi"("EncoderDevRef"=w3679) -> ("EncoderDevRef"=w3680:T11)  [unwired: 9 in, 1 out]
                          n1066 = Wait (ms)(milliseconds to wait=u32 10) -> ()  [unwired: 1 out]
                          n1067 = call <vilib>:"WPI_EncoderReset.vi"("EncoderDevRef"=w3678) -> ("EncoderDevRef"=w3681:T11)  [unwired: 9 in, 1 out]
                        }
                        frame #2 {
                          n1068 = global read "Robot Global Data.vi" "Axes"() -> (w3699:dbl[])
                          n1069 = Wait (ms)(milliseconds to wait=u32 400) -> ()  [unwired: 1 out]
                          n1070 = Array To Cluster(array=w3699) -> (cluster=w3700:T15)
                          n1071 = global read "Robot Global Data.vi" "PIXY Output"() -> (w3689:T16)
                          n1072 = Bundle By Name(cluster=w3700, "Axes[1]"=1.0) -> (w3701:T15)
                          n1073 = Unbundle By Name(w3689) -> ("SIGNATURE NUMBER"=w3696:u16)
                          n1074 = global read "Robot Global Data.vi" "Cube Signature"() -> (w3694:dbl)
                          n1075 = Equal?(x=w3696, y=w3694) -> (x = y?=w3695:bool)
                          n1076 = Cluster To Array(cluster=w3701) -> (array=w3702:dbl[])
                          n1077 = global write "Robot Global Data.vi" "Axes"(w3702) -> ()
                          n1078 = case shown="True" w3695 {
                            tunnel: [w3704 w3717] -> w3687
                            tunnel: [w3703 w3716] -> w3686
                            tunnel: [w3706 w3715] -> w3688
                            tunnel: [w3707 w3714] -> w3685
                            tunnel: w3693 -> [w3705 w3711]
                            tunnel: w3692 -> [w3706 w3710]
                            tunnel: w3691 -> [w3703 w3709]
                            tunnel: w3690 -> [w3704 w3708]
                            frame True {
                              n1079 = call "PID vision.vi"("RobotDriveDevRef in"=w3705) -> ("RobotDriveDevRef out"=w3707:T1)  [unwired: 9 in, 1 out]
                            }
                            frame False {
                              n1080 = call "PID Distance.vi"("Distance"=45.0, "Angle"=170.0, "RightEncoder"=w3708, "LeftEncoder"=w3709, "GyroDevRef"=w3710, "RobotDriveDevRef"=w3711) -> ("RightEncoder 2"=w3717:T11, "LeftEncoder 2"=w3716:T11, "GyroDevRef 2"=w3715:T8, "RobotDriveDevRef 2"=w3714:T1)  [unwired: 2 in]
                            }
                          }
                        }
                        frame #3 {
                          n1081 = call <vilib>:"WPI_EncoderReset.vi"("EncoderDevRef"=w3723) -> ("EncoderDevRef"=w3719:T11)  [unwired: 9 in, 1 out]
                          n1082 = call <vilib>:"WPI_EncoderReset.vi"("EncoderDevRef"=w3722) -> ("EncoderDevRef"=w3718:T11)  [unwired: 9 in, 1 out]
                          n1083 = Wait (ms)(milliseconds to wait=u32 10) -> ()  [unwired: 1 out]
                          n1084 = call <vilib>:"WPI_GyroGetAngle.vi"("GyroDevRef"=w3725) -> ("Angle"=w3724:dbl, "GyroDevRef"=w3720:T8)  [unwired: 6 in, 3 out]
                        }
                        frame #4 {
                          n1085 = call "PID with Infrared.vi"("RobotDriveDevRef"=w3731, "Angle"=w3733, "Encoder Limit"=20.0, "GyroDevRef"=w3730, "Left Encoder"=w3729, "Right Encoder"=w3728, "DigitalInputDevRef"=w3727) -> ()  [unwired: 4 in, 5 out]
                        }
                        frame #5 {
                          n1086 = global write "Robot Global Data.vi" "Current State"(TRUE ("Current State")) -> ()
                          n1087 = Wait (ms)(milliseconds to wait=u32 300) -> ()  [unwired: 1 out]
                        }
                      }
                    }
                    frame "R" {
                      n1088 = flat-sequence {
                        tunnel: w3763 -> [w3766]
                        tunnel: w3762 -> [w3765]
                        tunnel: [w3768] -> w3761
                        tunnel: [w3767] -> w3760
                        tunnel: w3761 -> [w3776]
                        tunnel: w3760 -> [w3775]
                        tunnel: w3759 -> [w3773]
                        tunnel: w3758 -> [w3772]
                        tunnel: [w3776] -> w3757
                        tunnel: [w3775] -> w3756
                        tunnel: [w3771] -> w3755
                        tunnel: [w3770] -> w3754
                        tunnel: [w3794] -> w3745
                        tunnel: [w3793] -> w3743
                        tunnel: [w3792] -> w3741
                        tunnel: [w3791] -> w3739
                        tunnel: w3754 -> [w3783]
                        tunnel: w3755 -> [w3784]
                        tunnel: w3756 -> [w3782]
                        tunnel: w3757 -> [w3781]
                        tunnel: w3745 -> [w3809]
                        tunnel: [w3808] -> w3744
                        tunnel: w3743 -> [w3811]
                        tunnel: [w3810] -> w3742
                        tunnel: w3741 -> [w3816]
                        tunnel: [w3814] -> w3740
                        tunnel: w3739 -> [w3817]
                        tunnel: [w3815] -> w3738
                        tunnel: w3737 -> [w3812]
                        tunnel: w3744 -> [w3823]
                        tunnel: w3742 -> [w3822]
                        tunnel: w3740 -> [w3821]
                        tunnel: w3738 -> [w3820]
                        tunnel: [w3823] -> w3753
                        tunnel: [w3822] -> w3751
                        tunnel: [w3821] -> w3749
                        tunnel: [w3820] -> w3747
                        tunnel: w3753 -> [w3832]
                        tunnel: [w3831] -> w3752
                        tunnel: w3751 -> [w3829]
                        tunnel: [w3830] -> w3750
                        tunnel: w3749 -> [w3841]
                        tunnel: [w3841] -> w3748
                        tunnel: w3747 -> [w3840]
                        tunnel: [w3840] -> w3746
                        tunnel: [w3824] -> w3736
                        tunnel: w3752 -> [w3846]
                        tunnel: w3750 -> [w3849]
                        tunnel: w3748 -> [w3848]
                        tunnel: w3746 -> [w3847]
                        tunnel: w3736 -> [w3843]
                        frame #0 {
                          n1089 = call "PID turning.vi"("Angle"=-170.0, "GyroDevRef"=w3765, "RobotDriveDevRef"=w3766) -> ("GyroDevRef 2"=w3767:T8, "RobotDriveDevRef 2"=w3768:T1)  [unwired: 7 in]
                        }
                        frame #1 {
                          n1090 = call <vilib>:"WPI_EncoderReset.vi"("EncoderDevRef"=w3772) -> ("EncoderDevRef"=w3770:T11)  [unwired: 9 in, 1 out]
                          n1091 = global write "Robot Global Data.vi" "Lift_Position"(0.0) -> ()
                          n1092 = Wait (ms)(milliseconds to wait=u32 10) -> ()  [unwired: 1 out]
                          n1093 = call <vilib>:"WPI_EncoderReset.vi"("EncoderDevRef"=w3773) -> ("EncoderDevRef"=w3771:T11)  [unwired: 9 in, 1 out]
                        }
                        frame #2 {
                          n1094 = global read "Robot Global Data.vi" "Axes"() -> (w3787:dbl[])
                          n1095 = Wait (ms)(milliseconds to wait=u32 400) -> ()  [unwired: 1 out]
                          n1096 = Array To Cluster(array=w3787) -> (cluster=w3788:T15)
                          n1097 = Bundle By Name(cluster=w3788, "Axes[1]"=1.0) -> (w3789:T15)
                          n1098 = global read "Robot Global Data.vi" "PIXY Output"() -> (w3777:T16)
                          n1099 = Unbundle By Name(w3777) -> ("SIGNATURE NUMBER"=w3780:u16)
                          n1100 = global read "Robot Global Data.vi" "Cube Signature"() -> (w3778:dbl)
                          n1101 = Equal?(x=w3780, y=w3778) -> (x = y?=w3779:bool)
                          n1102 = Cluster To Array(cluster=w3789) -> (array=w3790:dbl[])
                          n1103 = global write "Robot Global Data.vi" "Axes"(w3790) -> ()
                          n1104 = case shown="False" w3779 {
                            tunnel: [w3798 w3802] -> w3794
                            tunnel: [w3797 w3803] -> w3793
                            tunnel: [w3796 w3804] -> w3792
                            tunnel: [w3800 w3805] -> w3791
                            tunnel: w3784 -> [w3797 w3803]
                            tunnel: w3783 -> [w3798 w3802]
                            tunnel: w3782 -> [w3799 w3804]
                            tunnel: w3781 -> [w3801 w3805]
                            frame True {
                              n1105 = call <vilib>:"WPI_GyroGetAngle.vi"("GyroDevRef"=w3799) -> ("Angle"=w3795:dbl, "GyroDevRef"=w3796:T8)  [unwired: 6 in, 3 out]
                              n1106 = global write "Robot Global Data.vi" "Tracked Angle"(w3795) -> ()
                              n1107 = call "PID vision.vi"("RobotDriveDevRef in"=w3801) -> ("RobotDriveDevRef out"=w3800:T1)  [unwired: 9 in, 1 out]
                            }
                            frame False {
                              n1108 = global write "Robot Global Data.vi" "Tracked Angle"(-170.0) -> ()
                            }
                          }
                        }
                        frame #3 {
                          n1109 = global read "Robot Global Data.vi" "Tracked Angle"() -> (w3813:dbl)
                          n1110 = call "PID with Infrared.vi"("RobotDriveDevRef"=w3817, "Angle"=w3813, "Encoder Limit"=50.0, "GyroDevRef"=w3816, "Left Encoder"=w3811, "Right Encoder"=w3809, "DigitalInputDevRef"=w3812) -> ("RobotDriveDevRef 2"=w3815:T1, "GyroDevRef 2"=w3814:T8, "Left Encoder 2"=w3810:T11, "Right Encoder 2"=w3808:T11)  [unwired: 4 in, 1 out]
                        }
                        frame #4 {
                          n1111 = global write "Robot Global Data.vi" "Current State"(TRUE ("Current State")) -> ()
                          n1112 = Wait (ms)(milliseconds to wait=u32 500) -> ()  [unwired: 1 out]
                        }
                        frame #5 {
                          n1113 = global read "Robot Global Data.vi" "Axes"() -> (w3838:dbl[])
                          n1114 = global write "Robot Global Data.vi" "Lift_Position"(2.0) -> ()
                          n1115 = Wait (ms)(milliseconds to wait=u32 250) -> ()  [unwired: 1 out]
                          n1116 = Array To Cluster(array=w3838) -> (cluster=w3837:T15)
                          n1117 = Bundle By Name(cluster=w3837, "Axes[1]"=-1.0) -> (w3835:T15)
                          n1118 = call <vilib>:"WPI_EncoderGet.vi"("EncoderDevRef"=w3829) -> ("Distance"=w3828:dbl, "EncoderDevRef"=w3830:T11)  [unwired: 5 in, 4 out]
                          n1119 = call <vilib>:"WPI_EncoderGet.vi"("EncoderDevRef"=w3832) -> ("Distance"=w3827:dbl, "EncoderDevRef"=w3831:T11)  [unwired: 5 in, 4 out]
                          n1120 = Add(x=w3828, y=w3827) -> (x+y=w3826:dbl)
                          n1121 = Cluster To Array(cluster=w3835) -> (array=w3834:dbl[])
                          n1122 = global write "Robot Global Data.vi" "Axes"(w3834) -> ()
                          n1123 = Divide(x=w3826, y=2.0) -> (x/y=w3824:dbl)
                        }
                        frame #6 {
                          n1124 = Add(x=w3843, y=15.0 ("Distance")) -> (x+y=w3842:dbl)
                          n1125 = global read "Robot Global Data.vi" "Tracked Angle"() -> (w3845:dbl)
                          n1126 = call "PID Distance.vi"("Distance"=w3842, "Angle"=w3845, "RightEncoder"=w3846, "LeftEncoder"=w3849, "GyroDevRef"=w3848, "RobotDriveDevRef"=w3847) -> ()  [unwired: 2 in, 4 out]
                        }
                        frame #7 {
                          n1127 = global read "Robot Global Data.vi" "Axes"() -> (w3855:dbl[])
                          n1128 = Wait (ms)(milliseconds to wait=u32 250) -> ()  [unwired: 1 out]
                          n1129 = Array To Cluster(array=w3855) -> (cluster=w3854:T15)
                          n1130 = Bundle By Name(cluster=w3854, "Axes[1]"=1.0) -> (w3852:T15)
                          n1131 = Cluster To Array(cluster=w3852) -> (array=w3851:dbl[])
                          n1132 = global write "Robot Global Data.vi" "Axes"(w3851) -> ()
                        }
                        frame #8 {
                          n1133 = global write "Robot Global Data.vi" "Current State"(FALSE ("Current State")) -> ()
                        }
                      }
                    }
                    frame Default {
                    }
                  }
                }
              }
            }
            frame "L" {
              n1134 = flat-sequence {
                tunnel: [w3923] -> w3911
                tunnel: [w3922] -> w3912
                tunnel: [w3920] -> w3913
                tunnel: [w3921] -> w3914
                tunnel: w3870 -> [w3919]
                tunnel: w3869 -> [w3918]
                tunnel: w3868 -> [w3917]
                tunnel: w3867 -> [w3916]
                tunnel: [w3944] -> w3910
                tunnel: w3914 -> [w3940]
                tunnel: w3913 -> [w3941]
                tunnel: w3912 -> [w3943]
                tunnel: w3911 -> [w3945]
                tunnel: [w3942] -> w3909
                tunnel: [w3941] -> w3908
                tunnel: [w3940] -> w3907
                tunnel: w3910 -> [w3955]
                tunnel: [w3955] -> w3906
                tunnel: w3909 -> [w3954]
                tunnel: [w3954] -> w3905
                tunnel: [w3953] -> w3904
                tunnel: [w3952] -> w3903
                tunnel: w3908 -> [w3950]
                tunnel: w3907 -> [w3949]
                tunnel: w3906 -> [w3961]
                tunnel: [w3959] -> w3902
                tunnel: w3905 -> [w3960]
                tunnel: [w3958] -> w3901
                tunnel: w3904 -> [w3963]
                tunnel: w3903 -> [w3962]
                tunnel: [w3957] -> w3900
                tunnel: [w3956] -> w3899
                tunnel: w3902 -> [w3970]
                tunnel: [w3969] -> w3898
                tunnel: [w3968] -> w3897
                tunnel: w3901 -> [w3968]
                tunnel: [w3967] -> w3896
                tunnel: w3900 -> [w3967]
                tunnel: [w3966] -> w3895
                tunnel: w3899 -> [w3966]
                tunnel: [w3981] -> w3894
                tunnel: w3898 -> [w3981]
                tunnel: [w3980] -> w3893
                tunnel: w3897 -> [w3980]
                tunnel: [w3979] -> w3892
                tunnel: w3896 -> [w3979]
                tunnel: [w3978] -> w3891
                tunnel: w3895 -> [w3978]
                tunnel: w3894 -> [w3986]
                tunnel: w3893 -> [w3987]
                tunnel: [w3987] -> w3890
                tunnel: [w3986] -> w3889
                tunnel: [w3985] -> w3888
                tunnel: w3892 -> [w3985]
                tunnel: [w3984] -> w3887
                tunnel: w3891 -> [w3984]
                tunnel: [w4000] -> w3886
                tunnel: w3890 -> [w4002]
                tunnel: w3889 -> [w4001]
                tunnel: w3888 -> [w3997]
                tunnel: w3887 -> [w3996]
                tunnel: [w3995] -> w3885
                tunnel: [w3994] -> w3884
                tunnel: [w3993] -> w3883
                tunnel: w3886 -> [w4009]
                tunnel: w3885 -> [w4008]
                tunnel: [w4007] -> w3865
                tunnel: w3884 -> [w4007]
                tunnel: [w4006] -> w3863
                tunnel: w3883 -> [w4006]
                tunnel: [w4005] -> w3861
                tunnel: [w4004] -> w3859
                tunnel: w3865 -> [w4016]
                tunnel: [w4012] -> w3864
                tunnel: w3863 -> [w4015]
                tunnel: [w4011] -> w3862
                tunnel: w3861 -> [w4018]
                tunnel: [w4014] -> w3860
                tunnel: w3859 -> [w4017]
                tunnel: [w4013] -> w3858
                tunnel: w3864 -> [w4044]
                tunnel: w3862 -> [w4043]
                tunnel: [w4041] -> w3882
                tunnel: w3860 -> [w4041]
                tunnel: [w4040] -> w3881
                tunnel: w3858 -> [w4040]
                tunnel: [w4039] -> w3880
                tunnel: [w4038] -> w3879
                tunnel: w3882 -> [w4055]
                tunnel: w3881 -> [w4053]
                tunnel: w3880 -> [w4048]
                tunnel: w3879 -> [w4046]
                tunnel: [w4054] -> w3878
                tunnel: [w4052] -> w3877
                tunnel: [w4047] -> w3876
                tunnel: [w4045] -> w3875
                tunnel: w3857 -> [w4050]
                tunnel: [w4065] -> w3874
                tunnel: [w4062] -> w3873
                tunnel: [w4064] -> w3872
                tunnel: [w4063] -> w3871
                tunnel: w3875 -> [w4062]
                tunnel: w3876 -> [w4063]
                tunnel: w3877 -> [w4064]
                tunnel: w3878 -> [w4065]
                tunnel: w3874 -> [w4072]
                tunnel: w3873 -> [w4071]
                tunnel: w3872 -> [w4070]
                tunnel: w3871 -> [w4069]
                tunnel: w3866 -> [w4068]
                frame #0 {
                  n1135 = while {
                    tunnel: [w3929] -> w3915
                    stop <- w3928 stop-if-true
                    w3932 = 100.0 ("y")
                    w3935 = 20.0 ("y")
                    n1136 = Wait (ms)(milliseconds to wait=u32 10) -> ()  [unwired: 1 out]
                    n1137 = global read "Robot Global Data.vi" "Distance 2"() -> (w3930:dbl)
                    n1138 = global read "Robot Global Data.vi" "Distance"() -> (w3931:dbl)
                    n1139 = Greater?(x=w3931, y=w3935) -> (0:w3937:bool)
                    n1140 = Greater?(x=w3930, y=w3935) -> (0:w3936:bool)
                    n1141 = Greater?(x=w3931, y=w3932) -> (0:w3934:bool)
                    n1142 = Greater?(x=w3930, y=w3932) -> (0:w3933:bool)
                    n1143 = Or(x=w3937, y=w3936) -> (x .or. y?=w3926:bool)
                    n1144 = Or(x=w3934, y=w3933) -> (x .or. y?=w3928:bool)
                    n1145 = global write "Robot Global Data.vi" "Raise_Mast"(w3926) -> ()
                    n1146 = case shown="True" w3928 {
                      tunnel: [0.0 2.0] -> w3929
                      frame False {
                      }
                      frame True {
                      }
                    }
                  }
                  n1147 = call "PID Distance.vi"("Distance"=295.0, "Angle"=-2.0, "RightEncoder"=w3916, "LeftEncoder"=w3917, "GyroDevRef"=w3918, "RobotDriveDevRef"=w3919) -> ("RightEncoder 2"=w3920:T11, "LeftEncoder 2"=w3921:T11, "GyroDevRef 2"=w3922:T8, "RobotDriveDevRef 2"=w3923:T1)  [unwired: 2 in]
                  n1148 = global write "Robot Global Data.vi" "Lift_Position"(w3915) -> ()
                }
                frame #1 {
                  n1149 = call "PID turning.vi"("Angle"=90.0, "GyroDevRef"=w3943, "RobotDriveDevRef"=w3945) -> ("GyroDevRef 2"=w3942:T8, "RobotDriveDevRef 2"=w3944:T1)  [unwired: 7 in]
                  n1150 = global write "Robot Global Data.vi" "Lift_Position"(3.0) -> ()
                  n1151 = global write "Robot Global Data.vi" "Raise_Mast"(TRUE ("Current State")) -> ()
                }
                frame #2 {
                  n1152 = call <vilib>:"WPI_EncoderReset.vi"("EncoderDevRef"=w3949) -> ("EncoderDevRef"=w3952:T11)  [unwired: 9 in, 1 out]
                  n1153 = Wait (ms)(milliseconds to wait=u32 100) -> ()  [unwired: 1 out]
                  n1154 = call <vilib>:"WPI_EncoderReset.vi"("EncoderDevRef"=w3950) -> ("EncoderDevRef"=w3953:T11)  [unwired: 9 in, 1 out]
                }
                frame #3 {
                  n1155 = call "PID Distance.vi"("Distance"=25.0, "Angle"=90.0, "RightEncoder"=w3963, "LeftEncoder"=w3962, "GyroDevRef"=w3960, "RobotDriveDevRef"=w3961) -> ("RightEncoder 2"=w3956:T11, "LeftEncoder 2"=w3957:T11, "GyroDevRef 2"=w3958:T8, "RobotDriveDevRef 2"=w3959:T1)  [unwired: 2 in]
                }
                frame #4 {
                  w3971 = 0.0 ("Left axis value")
                  n1156 = global read "Robot Global Data.vi" "Axes"() -> (w3974:dbl[])
                  n1157 = Wait (ms)(milliseconds to wait=u32 500) -> ()  [unwired: 1 out]
                  n1158 = Array To Cluster(array=w3974) -> (cluster=w3973:T15)
                  n1159 = Bundle By Name(cluster=w3973, "Axes[1]"=0.25) -> (w3976:T15)
                  n1160 = Cluster To Array(cluster=w3976) -> (array=w3975:dbl[])
